vi "ClassPanel.vi"(8 "error in (no error)":errorcluster caption="entrée d'erreur (pas d'erreur)", 11 "TaikoLaser.lvclass":refnum<class "TaikoLaser.lvclass">) -> (0 "error out":errorcluster caption="sortie d'erreur", 3 "TaikoLaser.lvclass Out":refnum<class "TaikoLaser.lvclass">)   [LabVIEW 2019, in "TaikoLaser.lvclass"]
uses:
  TaikoLaser.lvclass
  <userlib>/TaikoLaser/PDLM_LaserMode.ctl
  C:/Programmes Labview/LabscanV1A/DevicesClass/BaseDevice/BaseDevice.lvclass
  <userlib>/TaikoLaser/PDLM_Tag.ctl
  <userlib>/TaikoLaser/PDLM_SystemStatus.ctl
  <userlib>/TaikoLaser/PDLM_TaggedValueList.ctl
  <userlib>/TaikoLaser/PDLM_TaggedValue.ctl
  TaikoLaser.lvclass/TaikoLaser.ctl
  BaseDevice/ClassQueueMess.ctl
  BaseDevice/BaseDevice.lvclass/BaseDevice.ctl
  <userlib>/TaikoLaser/PDLM_LaserLock.ctl
  BaseDevice/Accessor/GetBaseDataPath.vi
  BaseDevice/Accessor/GetClassEvent.vi
  <vilib>/Utility/error.llb/Error Cluster From Error Code.vi
  <vilib>/ErrorRing/Error Ring.xnode
panel:
  out "Error string":string
  out "ForceDis":bool caption="Force disconnect"
  out "Error":bool
  in  "UpdateCnter":u32
  out "JournalPath":path
  in  "Con/Disc.":bool
  out "InfoStr":string
  out "Shape String":string caption="Pulse Shape"
  out "Interlock":bool
  out "Temp":dbl caption="Temp (C)" min=0.1 step=0.1 format="%#.1f"
  out "updatedTag":T1[](array[typedef]) format="%x" items=["NONE"=0, "Locked"=16, "SoftLock"=17, "KeyLock"=18, "Class_IV_Lock"=20, "Interlock"=24, "LaserMode"=32, "LDH_PulsePowerTable"=33, "TriggerMode"=48, "TriggerLevelRaw"=64, "TriggerLevelRawLoLimit"=65, "TriggerLevelRawHiLimit"=66, "TriggerLevel"=72, "TriggerLevelLoLimit"=73, "TriggerLevelHiLimit"=74, "FastGate"=80, "FastGateImp"=96, "SlowGate"=112, "TargetTempRaw"=144, "TargetTempRawLoLimit"=145, "TargetTempRawHiLimit"=146, "CurrentTempRaw"=148, "CaseTempRaw"=149, "TargetTemp"=152, "TargetTempLoLimit"=153, "TargetTempHiLimit"=154, "CurrentTemp"=156, "CaseTemp"=157, "TempScale"=159, "Frequency"=168, "FrequencyLoLimit"=169, "FrequencyHiLimit"=170, "PulsePowerRaw"=176, "PulsePowerRawLoLimit"=177, "PulsePowerRawHiLimit"=178, "PulsePowerPermille"=180, "PulseShape"=181, "PulsePower"=184, "PulsePowerLoLimit"=185, "PulsePowerHiLimit"=186, "PulsePowerNanowatt"=188, "PulsePowerVoltage"=190, "PulseEnergy"=191, "CwPowerRaw"=192, "CwPowerRawLoLimit"=193, "CwPowerRawHiLimit"=194, "CwPowerPermille"=196, "CwPower"=200, "CwPowerLoLimit"=201, "CwPowerHiLimit"=202, "CwPowerMicroWatt"=204, "BurstLen"=208, "BurstPeriod"=224, "LDH_Fan"=240, "UI_Exclusive"=256]
  out "Act Power":dbl caption="Act. Power (mW)" min=0.1 step=0.1 format="%#.3f"
  in  "Update":bool
  in  "LaserMode":T2 caption="Laser Mode"
  in  "SoftLock":bool
  out "OnOffLock":bool
  out "KeyLock":bool
  in  "Power":dbl=0.1 caption="Output Power(%)" min=0.1 max=100.0 step=0.1 format="%#.1f"
  in  "MainProgQ":refnum<queue>
  in  "MainProgQEvent":refnum<user-event>
  in  "Acq":bool
  in  "Stop":bool
  in  "Frequ":dbl=50000.0 caption="Output Freq(kHz)" min=1.0 max=100000000.0 step=0.1 format="%#.1f"
  out "Init Program":bool
  # "Taiko Laser"
  # "this MUST labeled with class name"
  # "this MUST be present and labeled \"Stop\" and \"Acq\""
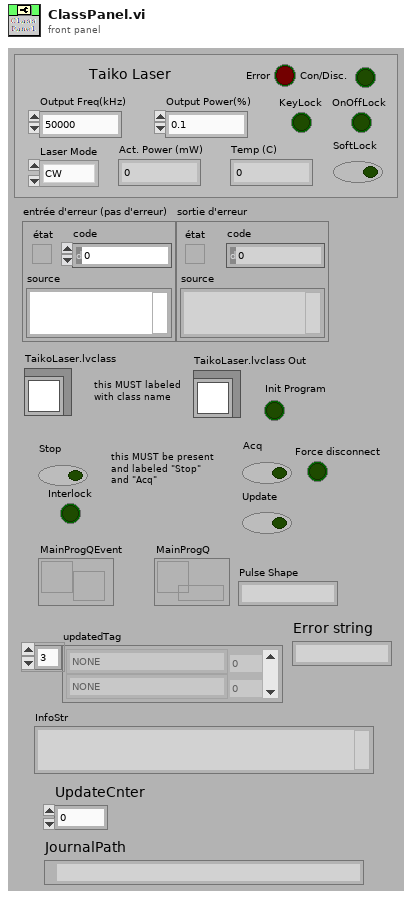
[diagram p1: front panel]
types:
  T1 = typedef "PDLM_Tag.ctl" = u32
  T2 = typedef "PDLM_LaserMode.ctl" = enum32{"CW", "PULSE", "BURST"}
  T3 = typedef "PDLM_SystemStatus.ctl" = u32
  T4 = typedef "PDLM_LaserLock.ctl" = enum32{"UNLOCKED", "LOCKED"}
  T5 = typedef "PDLM_TaggedValue.ctl" = cluster{"Tag":T1, "Value":u32}
  T6 = typedef "PDLM_TaggedValueList.ctl" = T5[]
  T7 = typedef "ClassQueueMess.ctl" = u16
  T8 = typedef "PDLM_LHInfo.ctl" = cluster{"LType":string, "Date":string, "LClass":string}
  T9 = typedef "PDLM_LHData.ctl" = cluster{"SerNo":u32, "Features":u32, "FreqMin":u32, "FreqMax":u32, "CwPowerMax":u32, "PulsePowerMax":u32, "WavelengthNominal":u16, "CaseTempMax":u16, "Protection":bool, "LHTypeCtrlVoltage":u16, "LHMaxVoltage":u16, "CurrentTEP12V":u16, "LaserType":T10, "LHVersion":T11, "CalWarrentHours":u16}
  T10 = typedef "PDLM_LHData_LaserType.ctl" = u16
  T11 = typedef "PDLM_LHVersion.ctl" = cluster{"Major":u16, "Minor":u16}
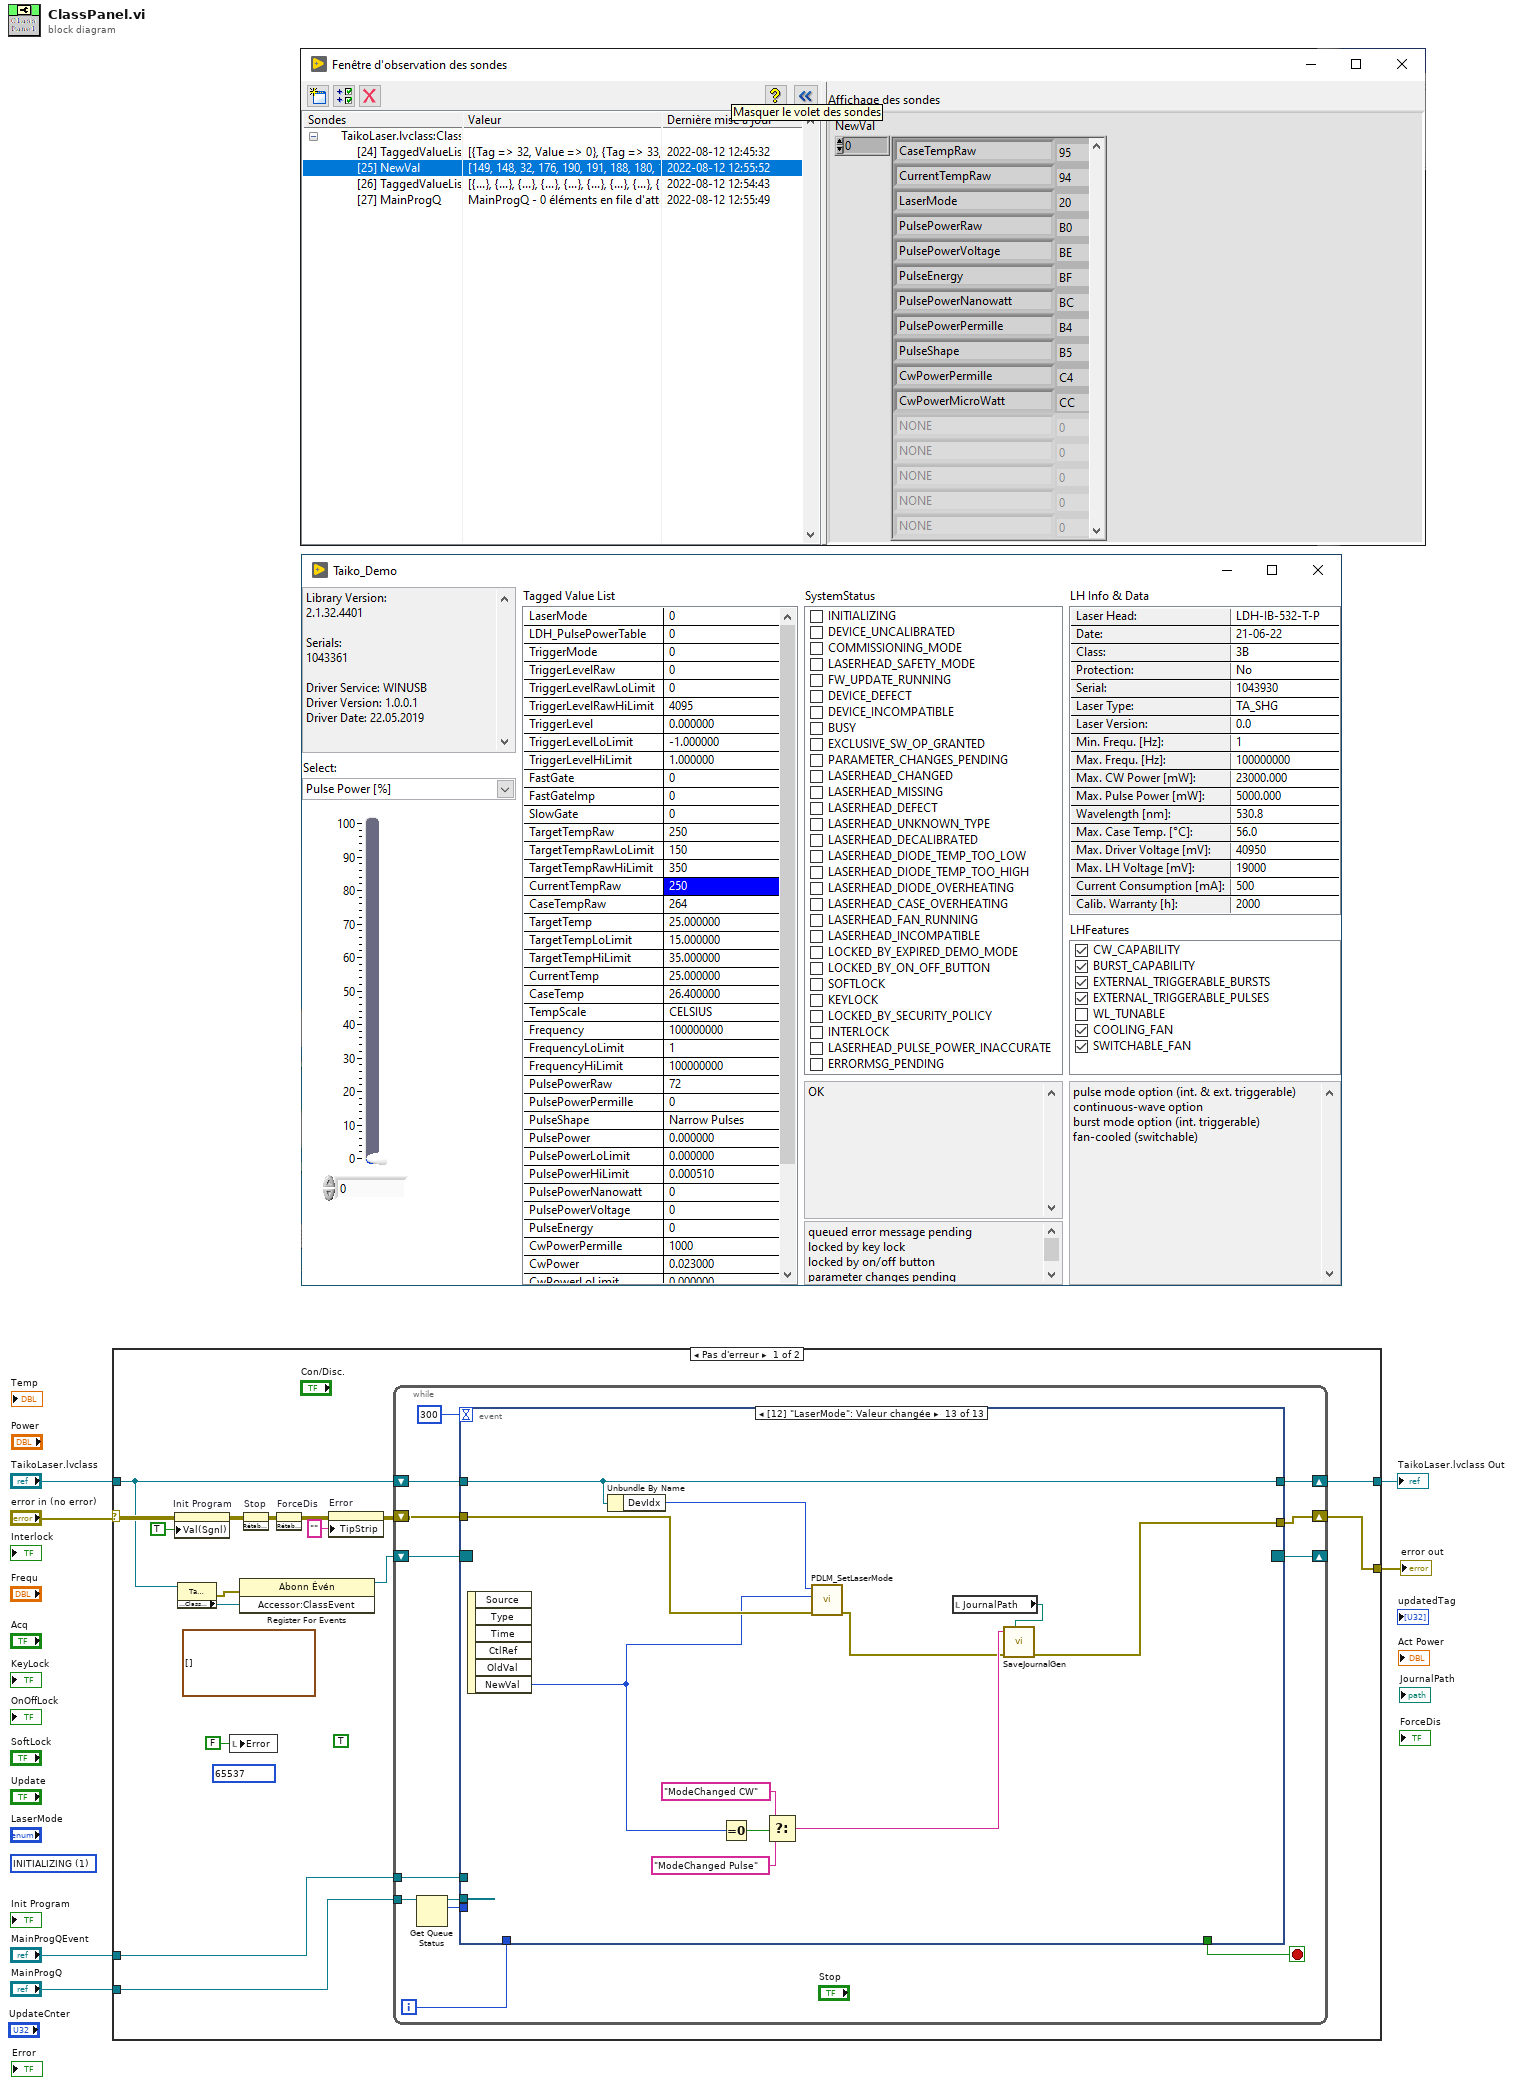
[diagram p0: block diagram]
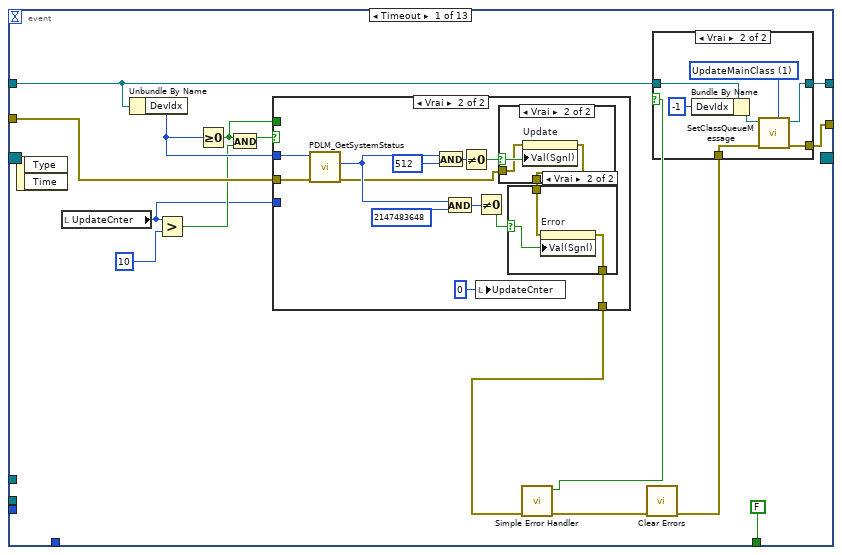
[diagram p2: hidden frame]
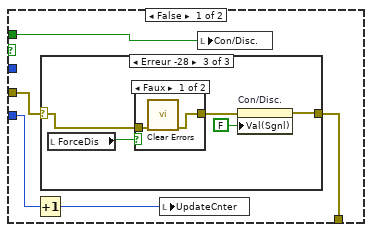
[diagram p4: hidden frame]
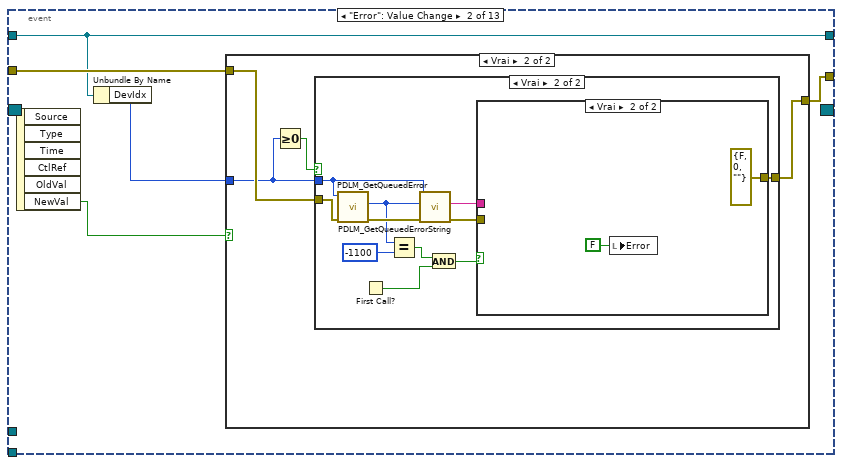
[diagram p10: hidden frame]
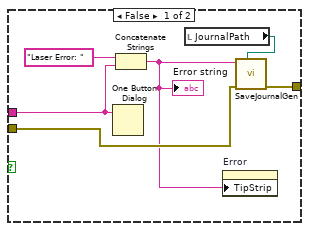
[diagram p13: hidden frame]
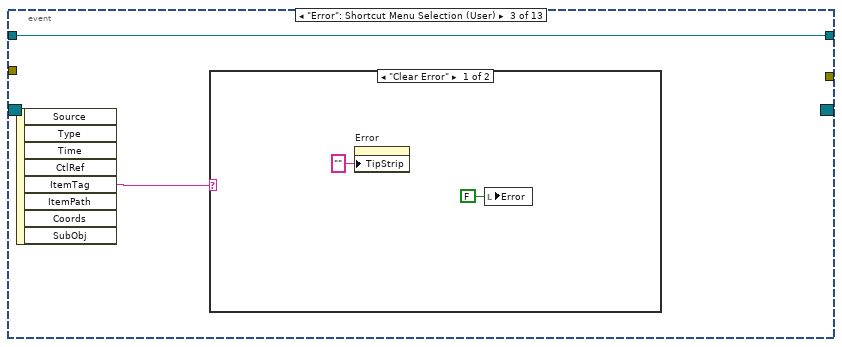
[diagram p14: hidden frame]
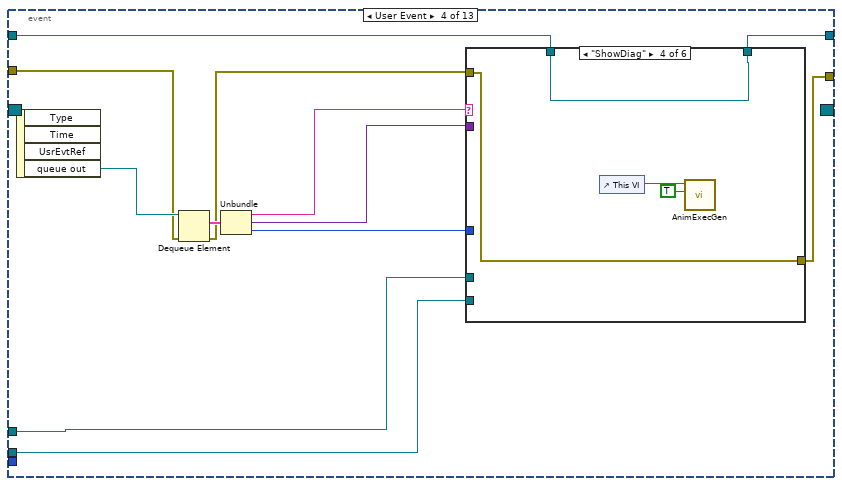
[diagram p16: hidden frame]
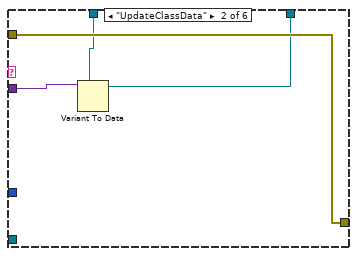
[diagram p18: hidden frame]
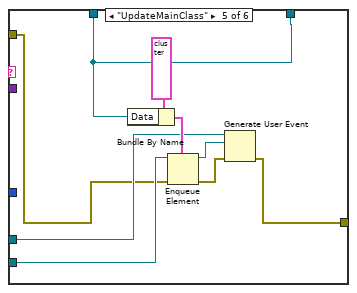
[diagram p20: hidden frame]
diagram:
  (unwired) T3 1 items=["INITIALIZING"=1, "DEVICE_UNCALIBRATED"=2, "COMMISSIONING_MODE"=4, "LASERHEAD_SAFETY_MODE"=8, "FW_UPDATE_RUNNING"=16, "DEVICE_DEFECT"=32, "DEVICE_INCOMPATIBLE"=64, "BUSY"=128, "EXCLUSIVE_SW_OP_GRANTED"=256, "PARAMETER_CHANGES_PENDING"=512, "LASERHEAD_CHANGED"=2048, "LASERHEAD_MISSING"=4096, "LASERHEAD_DEFECT"=8192, "LASERHEAD_UNKNOWN_TYPE"=16384, "LASERHEAD_DECALIBRATED"=32768, "LASERHEAD_DIODE_TEMP_TOO_LOW"=65536, "LASERHEAD_DIODE_TEMP_TOO_HIGH"=131072, "LASERHEAD_DIODE_OVERHEATING"=262144, "LASERHEAD_CASE_OVERHEATING"=524288, "LASERHEAD_FAN_RUNNING"=1048576, "LASERHEAD_INCOMPATIBLE"=2097152, "LOCKED_BY_EXPIRED_DEMO_MODE"=4194304, "LOCKED_BY_ON_OFF_BUTTON"=8388608, "SOFTLOCK"=16777216, "KEYLOCK"=33554432, "LOCKED_BY_SECURITY_POLICY"=67108864, "INTERLOCK"=134217728, "LASERHEAD_PULSE_POWER_INACCURATE"=268435456, "ERRORMSG_PENDING"=2147483648] ("SystemStatus")
  n1 = case shown="Pas d'erreur" "error in (no error)" {
    selector: "error in (no error)" -> [w11 w565]
    tunnel: [w22 w565] -> w5
    tunnel: "TaikoLaser.lvclass" -> [w16 w564]
    tunnel: [w20 w564] -> w3
    tunnel: "MainProgQEvent" -> [w14 _]
    tunnel: "MainProgQ" -> [w13 _]
    frame No Error {
      (unwired) TRUE ("ForceDis")
      (unwired) T1 65537 items=["NONE"=0, "Locked"=16, "SoftLock"=17, "KeyLock"=18, "Class_IV_Lock"=20, "Interlock"=24, "LaserMode"=32, "LDH_PulsePowerTable"=33, "TriggerMode"=48, "TriggerLevelRaw"=64, "TriggerLevelRawLoLimit"=65, "TriggerLevelRawHiLimit"=66, "TriggerLevel"=72, "TriggerLevelLoLimit"=73, "TriggerLevelHiLimit"=74, "FastGate"=80, "FastGateImp"=96, "SlowGate"=112, "TargetTempRaw"=144, "TargetTempRawLoLimit"=145, "TargetTempRawHiLimit"=146, "CurrentTempRaw"=148, "CaseTempRaw"=149, "TargetTemp"=152, "TargetTempLoLimit"=153, "TargetTempHiLimit"=154, "CurrentTemp"=156, "CaseTemp"=157, "TempScale"=159, "Frequency"=168, "FrequencyLoLimit"=169, "FrequencyHiLimit"=170, "PulsePowerRaw"=176, "PulsePowerRawLoLimit"=177, "PulsePowerRawHiLimit"=178, "PulsePowerPermille"=180, "PulseShape"=181, "PulsePower"=184, "PulsePowerLoLimit"=185, "PulsePowerHiLimit"=186, "PulsePowerNanowatt"=188, "PulsePowerVoltage"=190, "PulseEnergy"=191, "CwPowerRaw"=192, "CwPowerRawLoLimit"=193, "CwPowerRawHiLimit"=194, "CwPowerPermille"=196, "CwPower"=200, "CwPowerLoLimit"=201, "CwPowerHiLimit"=202, "CwPowerMicroWatt"=204, "BurstLen"=208, "BurstPeriod"=224, "LDH_Fan"=240, "UI_Exclusive"=256] ("Tag")
      (unwired) T6 [] ("TaggedValueList")
      n2 = property on="Init Program" class="Bool (strict)"(error in=w11, "Val(Sgnl)"=TRUE ("Valeur (Signalisation)")) -> (error out=w19:errorcluster)  [unwired: 1 in, 1 out]
      n3 = property class="TaikoLaser.lvclass"(reference=w16) -> (error out=w18:errorcluster, "Accessor:ClassEvent"=w17:refnum<user-event>)  [unwired: 1 in, 1 out]
      n4 = local write "Error"(FALSE ("Error")) -> ()
      n5 = register-events(error in=w18, w17) -> (reference out=w15:refnum<event-registration>)  [unwired: 1 in, 1 out]
      n6 = invoke on="Stop" class="Bool (strict)" method="RétablirValParDéfaut"(error in=w19) -> (error out=w10:errorcluster)  [unwired: 2 in, 2 out]
      n7 = invoke on="ForceDis" class="Bool (strict)" method="RétablirValParDéfaut"(error in=w10) -> (error out=w9:errorcluster)  [unwired: 2 in, 2 out]
      n8 = property on="Error" class="Bool (strict)"(error in=w9, "TipStrip"="" ("Info-bulle")) -> (error out=w8:errorcluster)  [unwired: 1 in, 1 out]
      n9 = while {
        shift-right: [w33] -> w22
        shift-left: w8 -> [w34]
        shift-right: [w32] -> w20
        shift-left: w16 -> [w26]
        shift-right: [w30] -> _
        shift-left: w15 -> [w31]
        tunnel: w14 -> [w29]
        tunnel: w13 -> [w28]
        i -> [w27]
        stop <- w25 stop-if-true
        n10 = Get Queue Status(queue=w28) -> (queue out=w24:refnum<queue>, # pending remove=w23:i32)  [unwired: 2 in, 6 out]
        n11 = event shown="[12] \"LaserMode\": Valeur changée" {
          selector: w31 -> [_ _ _ _ _ _ _ _ _ _ _ _ _]
          dyn-events: [_ _ _ _ _ _ _ _ _ _ _ _ _] -> w30
          timeout: 300 -> [_ _ _ _ _ _ _ _ _ _ _ _ _]
          tunnel: w34 -> [w48 w98 _ w131 w171 w208 w303 w317 w334 w354 w371 w415 w563]
          tunnel: [w42 w99 _ w135 w168 w213 w296 w313 w331 w345 w370 w409 w554] -> w33
          tunnel: w26 -> [w47 w97 w126 w141 w169 w211 w299 w316 w342 w357 w369 w412 w562]
          tunnel: [FALSE _ _ _ FALSE FALSE TRUE _ _ _ _ _ _] -> w25
          tunnel: [w45 w97 w126 w134 w167 w210 w299 w316 w342 w357 w368 w407 w562] -> w32
          tunnel: w29 -> [_ _ _ w133 _ _ _ _ _ _ _ _ _]
          tunnel: w24 -> [_ _ _ w132 _ _ _ _ _ _ _ _ _]
          tunnel: w27 -> [_ _ _ _ _ _ _ _ _ _ _ _ _]
          tunnel: w23 -> [_ _ _ _ _ _ _ _ _ _ _ _ _]
          event Timeout {
            n12 = event-data() -> ()  [unwired: 1 in, 2 out]
            n13 = local read "UpdateCnter"() -> (w38:u32)
            n14 = Unbundle By Name(w47) -> ("DevIdx"=w46:i32)
            n15 = Greater?(x=w38, y=u32 10) -> (0:w39:bool)
            n16 = Greater Or Equal To 0?(x=w46) -> (x >= 0?=w36:bool)
            n17 = And(x=w36, y=w39) -> (x .and. y?=w40:bool)
            n18 = case shown="Vrai" w40 {
              tunnel: w48 -> [w61 w87]
              tunnel: w46 -> [_ w86]
              tunnel: w38 -> [w64 _]
              tunnel: [w60 w75] -> w37
              tunnel: w36 -> [w62 _]
              frame False {
                n19 = Increment(x=w64) -> (x+1=w63:u32)
                n20 = case shown="Erreur -28" w61 {
                  selector: w61 -> [w65 w66 w70]
                  tunnel: [w65 w66 w68] -> w60
                  frame No Error {
                  }
                  frame Default {
                  }
                  frame Error {
                    n21 = local read "ForceDis"() -> (w71:bool)
                    n22 = case shown="Faux" w71 {
                      tunnel: w70 -> [w73 w74]
                      tunnel: [w72 w74] -> w69
                      frame False {
                        n23 = call <vilib>:"Clear Errors.vi"("error in (no error)"=w73) -> ("error out"=w72:errorcluster)  [unwired: 5 in, 1 out]
                      }
                      frame True {
                      }
                    }
                    n24 = property on="Con/Disc." class="Bool (strict)"(error in=w69, "Val(Sgnl)"=FALSE ("Valeur (Signalisation)")) -> (error out=w68:errorcluster)  [unwired: 1 in, 1 out]
                  }
                }
                n25 = local write "UpdateCnter"(w63) -> ()
                n26 = local write "Con/Disc."(w62) -> ()
              }
              frame True {
                n27 = call <userlib>:"PDLM_GetSystemStatus.vi"("error in (no error)"=w87, "USBIdx"=w86) -> ("error out"=w76:errorcluster, "state"=w82:u32)  [unwired: 7 in, 1 out]
                n28 = And(x=w82, y=u32 512) -> (x .and. y?=w81:u32)
                n29 = And(x=w82, y=u32 2147483648) -> (x .and. y?=w83:u32)
                n30 = Not Equal To 0?(x=w81) -> (x != 0?=w80:bool)
                n31 = Not Equal To 0?(x=w83) -> (x != 0?=w78:bool)
                n32 = local write "UpdateCnter"(u32 0 ("UpdateCnter")) -> ()
                n33 = case shown="Vrai" w80 {
                  selector: w80 -> [_ w95]
                  tunnel: [w92 w94] -> w77
                  tunnel: w76 -> [w92 w93]
                  frame False {
                  }
                  frame True {
                    n34 = property on="Update" class="Bool (strict)"(error in=w93, "Val(Sgnl)"=w95) -> (error out=w94:errorcluster)  [unwired: 1 in, 1 out]
                  }
                }
                n35 = case shown="Vrai" w78 {
                  selector: w78 -> [_ w91]
                  tunnel: w77 -> [w88 w90]
                  tunnel: [w88 w89] -> w75
                  frame False {
                  }
                  frame True {
                    n36 = property on="Error" class="Bool (strict)"(error in=w90, "Val(Sgnl)"=w91) -> (error out=w89:errorcluster)  [unwired: 1 in, 1 out]
                  }
                }
              }
            }
            n37 = call <vilib>:"Simple Error Handler.vi"("error in (no error)"=w37) -> ("error?"=w44:bool, "error out"=w49:errorcluster)  [unwired: 4 in, 3 out]
            n38 = call <vilib>:"Clear Errors.vi"("error in (no error)"=w49) -> ("error out"=w43:errorcluster)  [unwired: 5 in, 1 out]
            n39 = case shown="Vrai" w44 {
              tunnel: w47 -> [w52 w59]
              tunnel: [w52 w56] -> w45
              tunnel: w43 -> [w51 w54]
              tunnel: [w51 w53] -> w42
              frame False {
              }
              frame True {
                w55 = T7 1 items=["UpdateClassData", "UpdateMainClass", "UpdateDataBind"] ("Menu déroulant")
                n40 = Bundle By Name(cluster=w59, "DevIdx"=-1) -> (w57:refnum<class "TaikoLaser.lvclass">)
                n41 = call-dynamic "SetClassQueueMessage.vi"("ErrorIn(No Error)"=w54, "Menu déroulant"=w55, "DefaultDev.lvclass"=w57) -> ("sortie d'erreur"=w53:errorcluster, "DefaultDev.lvclass Out"=w56:refnum<class "TaikoLaser.lvclass">)  [unwired: 7 in]
              }
            }
          }
          event "Error": Value Change {
            n42 = event-data() -> ("NewVal"=w100:bool)  [unwired: 1 in, 5 out]
            n43 = Unbundle By Name(w97) -> ("DevIdx"=w96:i32)
            n44 = case shown="Vrai" w100 {
              tunnel: [w101 w104] -> w99
              tunnel: w98 -> [w101 w105]
              tunnel: w96 -> [_ w103]
              frame False {
              }
              frame True {
                n45 = Greater Or Equal To 0?(x=w103) -> (x >= 0?=w102:bool)
                n46 = case shown="Vrai" w102 {
                  tunnel: w103 -> [_ w116]
                  tunnel: w105 -> [w106 w115]
                  tunnel: [w106 w112] -> w104
                  frame False {
                  }
                  frame True {
                    n47 = call <userlib>:"PDLM_GetQueuedError.vi"("error in (no error)"=w115, "USBIdx"=w116) -> ("error out"=w117:errorcluster, "ErrCode"=w111:i32)  [unwired: 7 in, 1 out]
                    n48 = First Call?() -> (First Call?: T/F=w109:bool)
                    n49 = Equal?(x=w111, y=-1100) -> (x = y?=w108:bool)
                    n50 = call <userlib>:"PDLM_GetQueuedErrorString.vi"("error in (no error)"=w117, "ErrCode"=w111, "USBIdx"=w116) -> ("error out"=w113:errorcluster, "ErrText"=w114:string)  [unwired: 6 in, 1 out]
                    n51 = And(x=w108, y=w109) -> (x .and. y?=w107:bool)
                    n52 = case shown="Vrai" w107 {
                      tunnel: w114 -> [w122 _]
                      tunnel: w113 -> [w120 _]
                      tunnel: [w119 errorcluster {"status"=FALSE, "code"=0, "source"=""} ("error out")] -> w112
                      frame False {
                        n53 = One Button Dialog(message=w122) -> ()  [unwired: 1 in, 1 out]
                        n54 = Concatenate Strings("Laser Error: " ("chaîne"), w122) -> (w118:string)
                        "Error string" <- w118
                        n55 = local read "JournalPath"() -> (w123:path)
                        n56 = property on="Error" class="Bool (strict)"("TipStrip"=w118) -> ()  [unwired: 2 in, 2 out]
                        n57 = call <userlib>:"SaveJournalGen.vi"("CheminSauv"=w123, "error in"=w120, "Journal Text"=w118) -> ("error out"=w119:errorcluster)  [unwired: 7 in, 1 out]
                      }
                      frame True {
                        n58 = local write "Error"(FALSE ("Error")) -> ()
                      }
                    }
                  }
                }
              }
            }
          }
          event "Error": Shortcut Menu Selection (User) {
            n59 = event-data() -> ("ItemTag"=w127:string)  [unwired: 1 in, 7 out]
            n60 = case shown="\"Clear Error\"" w127 {
              frame "Clear Error" {
                n61 = property on="Error" class="Bool (strict)"("TipStrip"="" ("Info-bulle")) -> ()  [unwired: 2 in, 2 out]
                n62 = local write "Error"(FALSE ("Error")) -> ()
              }
              frame Default {
              }
            }
          }
          event User Event {
            n63 = event-data() -> ("queue out"=w139:refnum<queue>)  [unwired: 1 in, 3 out]
            n64 = Dequeue Element(queue=w139, error in (no error)=w131) -> (element=w140:cluster{"Message":string, "Data":variant, i32}, error out=w130:errorcluster)  [unwired: 1 in, 2 out]
            n65 = Unbundle(w140) -> ("Message"=w138:string, "Data"=w137:variant, w136:i32)
            n66 = case shown="\"ShowDiag\"" w138 {
              tunnel: w130 -> [w143 w147 w148 w152 w155 w165]
              tunnel: w137 -> [_ w146 _ _ _ _]
              tunnel: w141 -> [w142 w145 w149 w153 w158 w166]
              tunnel: [w142 w144 w149 w153 w158 w166] -> w134
              tunnel: [w143 w147 w148 w152 w154 w164] -> w135
              tunnel: w136 -> [_ _ _ _ _ _]
              tunnel: w133 -> [_ _ _ _ w157 _]
              tunnel: w132 -> [_ _ _ _ w156 _]
              frame Default {
              }
              frame "UpdateClassData" {
                n67 = Variant To Data(type=w145, Variant=w146) -> (data=w144:refnum<class "TaikoLaser.lvclass">)  [unwired: 1 in, 1 out]
              }
              frame "MeasDone" {
              }
              frame "ShowDiag" {
                n68 = control-ref of="This VI"() -> (w151:refnum<vi>)
                n69 = call <userlib>:"AnimExecGen.vi"("Animer l'exécution ?"=TRUE, "ViRef"=w151) -> ()  [unwired: 9 in, 1 out]
              }
              frame "UpdateMainClass" {
                n70 = Bundle By Name(cluster=cluster{"Message":string, "Data":variant, i32} {"Message"="", "Data"=variant, 0} ("élément"), "Data"=w158) -> (w159:cluster{"Message":string, "Data":variant, i32})
                n71 = Enqueue Element(queue=w156, element=w159, error in (no error)=w155) -> (queue out=w162:refnum<queue>, error out=w161:errorcluster)  [unwired: 1 in, 1 out]
                n72 = Generate User Event(user event=w157, event data cluster=w162, error in=w161) -> (error out=w154:errorcluster)  [unwired: 1 in, 1 out]
              }
              frame "ReInitDevice" {
                n73 = property on="Init Program" class="Bool (strict)"(error in=w165, "Val(Sgnl)"=TRUE ("Valeur (Signalisation)")) -> (error out=w164:errorcluster)  [unwired: 1 in, 1 out]
              }
            }
          }
          event "Con/Disc.": Value Change {
            n74 = event-data() -> ("NewVal"=w170:bool)  [unwired: 1 in]
            n75 = case shown="Faux" w170 {
              tunnel: w171 -> [w186 w204]
              tunnel: w169 -> [w182 w205]
              tunnel: [w178 w205] -> w167
              tunnel: [w177 w202] -> w168
              frame False {
                w180 = T7 1 items=["UpdateClassData", "UpdateMainClass", "UpdateDataBind"] ("Menu déroulant")
                n76 = Unbundle By Name(w182) -> ("DevIdx"=w185:i32)
                n77 = Greater Or Equal To 0?(x=w185) -> (x >= 0?=w184:bool)
                n78 = case shown="Faux" w184 {
                  tunnel: w186 -> [w191 w201]
                  tunnel: [w188 w200] -> w175
                  tunnel: w185 -> [_ w199]
                  tunnel: [w189 w198] -> w183
                  tunnel: w182 -> [w189 w198]
                  frame False {
                    n79 = local read "ForceDis"() -> (w187:bool)
                    n80 = case shown="Faux" w187 {
                      frame False {
                        n81 = property on="Init Program" class="Bool (strict)"("Val(Sgnl)"=TRUE ("Valeur (Signalisation)")) -> ()  [unwired: 2 in, 2 out]
                        n82 = local write "ForceDis"(TRUE ("ForceDis")) -> ()
                      }
                      frame True {
                      }
                    }
                    n83 = for {
                      N: 4 -> [_]
                      tunnel: w191 -> [w197]
                      tunnel: [w194] -> w188
                      tunnel: [w195] -> _
                      i -> [w196]
                      stop <- w194 continue-if-true
                      n84 = call <userlib>:"PDLM_CloseDevice.vi"("error in (no error)"=w197, "USBIdx"=w196) -> ("error out"=w194:errorcluster, "return type"=w195:i32)  [unwired: 8 in]
                    }
                  }
                  frame True {
                    n85 = call <userlib>:"PDLM_CloseDevice.vi"("error in (no error)"=w201, "USBIdx"=w199) -> ("error out"=w200:errorcluster)  [unwired: 8 in, 1 out]
                  }
                }
                n86 = Bundle By Name(cluster=w183, "DevIdx"=-1) -> (w179:refnum<class "TaikoLaser.lvclass">)
                n87 = local read "JournalPath"() -> (w176:path)
                n88 = call <userlib>:"SaveJournalGen.vi"("CheminSauv"=w176, "error in"=w175, "Journal Text"="TaikoSession Close") -> ("error out"=w174:errorcluster)  [unwired: 7 in, 1 out]
                n89 = call-dynamic "SetClassQueueMessage.vi"("ErrorIn(No Error)"=w174, "Menu déroulant"=w180, "DefaultDev.lvclass"=w179) -> ("sortie d'erreur"=w177:errorcluster, "DefaultDev.lvclass Out"=w178:refnum<class "TaikoLaser.lvclass">)  [unwired: 7 in]
              }
              frame True {
                n90 = property on="Init Program" class="Bool (strict)"(error in=w204, "Val(Sgnl)"=TRUE ("Valeur (Signalisation)")) -> (error out=w202:errorcluster)  [unwired: 1 in, 1 out]
              }
            }
          }
          event "Init Program": Value Change {
            n91 = event-data() -> ("NewVal"=w214:bool)  [unwired: 1 in]
            n92 = property class="TaikoLaser.lvclass"(reference=w211, error in=w208) -> (reference out=w209:refnum<class "TaikoLaser.lvclass">, error out=w207:errorcluster, "Accessor:BaseDataPath"=w206:path)
            n93 = case shown="Vrai" w214 {
              tunnel: w207 -> [w216 w232]
              tunnel: [w216 w248] -> w213
              tunnel: w209 -> [w215 w250]
              tunnel: [w215 w249] -> w210
              tunnel: w206 -> [_ w222]
              frame False {
              }
              frame True {
                w257 = T3 16777216 items=["INITIALIZING"=1, "DEVICE_UNCALIBRATED"=2, "COMMISSIONING_MODE"=4, "LASERHEAD_SAFETY_MODE"=8, "FW_UPDATE_RUNNING"=16, "DEVICE_DEFECT"=32, "DEVICE_INCOMPATIBLE"=64, "BUSY"=128, "EXCLUSIVE_SW_OP_GRANTED"=256, "PARAMETER_CHANGES_PENDING"=512, "LASERHEAD_CHANGED"=2048, "LASERHEAD_MISSING"=4096, "LASERHEAD_DEFECT"=8192, "LASERHEAD_UNKNOWN_TYPE"=16384, "LASERHEAD_DECALIBRATED"=32768, "LASERHEAD_DIODE_TEMP_TOO_LOW"=65536, "LASERHEAD_DIODE_TEMP_TOO_HIGH"=131072, "LASERHEAD_DIODE_OVERHEATING"=262144, "LASERHEAD_CASE_OVERHEATING"=524288, "LASERHEAD_FAN_RUNNING"=1048576, "LASERHEAD_INCOMPATIBLE"=2097152, "LOCKED_BY_EXPIRED_DEMO_MODE"=4194304, "LOCKED_BY_ON_OFF_BUTTON"=8388608, "SOFTLOCK"=16777216, "KEYLOCK"=33554432, "LOCKED_BY_SECURITY_POLICY"=67108864, "INTERLOCK"=134217728, "LASERHEAD_PULSE_POWER_INACCURATE"=268435456, "ERRORMSG_PENDING"=2147483648] ("SystemStatus")
                w264 = T3 33554432 items=["INITIALIZING"=1, "DEVICE_UNCALIBRATED"=2, "COMMISSIONING_MODE"=4, "LASERHEAD_SAFETY_MODE"=8, "FW_UPDATE_RUNNING"=16, "DEVICE_DEFECT"=32, "DEVICE_INCOMPATIBLE"=64, "BUSY"=128, "EXCLUSIVE_SW_OP_GRANTED"=256, "PARAMETER_CHANGES_PENDING"=512, "LASERHEAD_CHANGED"=2048, "LASERHEAD_MISSING"=4096, "LASERHEAD_DEFECT"=8192, "LASERHEAD_UNKNOWN_TYPE"=16384, "LASERHEAD_DECALIBRATED"=32768, "LASERHEAD_DIODE_TEMP_TOO_LOW"=65536, "LASERHEAD_DIODE_TEMP_TOO_HIGH"=131072, "LASERHEAD_DIODE_OVERHEATING"=262144, "LASERHEAD_CASE_OVERHEATING"=524288, "LASERHEAD_FAN_RUNNING"=1048576, "LASERHEAD_INCOMPATIBLE"=2097152, "LOCKED_BY_EXPIRED_DEMO_MODE"=4194304, "LOCKED_BY_ON_OFF_BUTTON"=8388608, "SOFTLOCK"=16777216, "KEYLOCK"=33554432, "LOCKED_BY_SECURITY_POLICY"=67108864, "INTERLOCK"=134217728, "LASERHEAD_PULSE_POWER_INACCURATE"=268435456, "ERRORMSG_PENDING"=2147483648] ("SystemStatus")
                w265 = T3 8388608 items=["INITIALIZING"=1, "DEVICE_UNCALIBRATED"=2, "COMMISSIONING_MODE"=4, "LASERHEAD_SAFETY_MODE"=8, "FW_UPDATE_RUNNING"=16, "DEVICE_DEFECT"=32, "DEVICE_INCOMPATIBLE"=64, "BUSY"=128, "EXCLUSIVE_SW_OP_GRANTED"=256, "PARAMETER_CHANGES_PENDING"=512, "LASERHEAD_CHANGED"=2048, "LASERHEAD_MISSING"=4096, "LASERHEAD_DEFECT"=8192, "LASERHEAD_UNKNOWN_TYPE"=16384, "LASERHEAD_DECALIBRATED"=32768, "LASERHEAD_DIODE_TEMP_TOO_LOW"=65536, "LASERHEAD_DIODE_TEMP_TOO_HIGH"=131072, "LASERHEAD_DIODE_OVERHEATING"=262144, "LASERHEAD_CASE_OVERHEATING"=524288, "LASERHEAD_FAN_RUNNING"=1048576, "LASERHEAD_INCOMPATIBLE"=2097152, "LOCKED_BY_EXPIRED_DEMO_MODE"=4194304, "LOCKED_BY_ON_OFF_BUTTON"=8388608, "SOFTLOCK"=16777216, "KEYLOCK"=33554432, "LOCKED_BY_SECURITY_POLICY"=67108864, "INTERLOCK"=134217728, "LASERHEAD_PULSE_POWER_INACCURATE"=268435456, "ERRORMSG_PENDING"=2147483648] ("SystemStatus")
                n94 = xnode "Menu déroulant d'erreurs"() -> ("sortie d'erreur"=w219:errorcluster)
                n95 = Not A Number/Path/Refnum?(number/path/refnum=w222) -> (NaN/Path/Refnum?=w225:bool)
                n96 = Empty String/Path?(string/path=w222) -> (empty?=w224:bool)
                n97 = call <userlib>:"PDLM_GetDLLPath.vi"("error in (no error)"=w232) -> ("error out"=w254:errorcluster)  [unwired: 8 in, 2 out]
                n98 = Or(x=w225, y=w224) -> (x .or. y?=w223:bool)
                n99 = for {
                  N: 8 -> [_]
                  tunnel: [w292] -> w251
                  tunnel: [w293] -> w218
                  tunnel: w254 -> [w294]
                  i -> [w292]
                  stop <- w293 continue-if-true
                  n100 = call <userlib>:"PDLM_OpenDevice.vi"("error in (no error)"=w294, "USBIdx"=w292) -> ("error out"=w293:errorcluster)  [unwired: 7 in, 2 out]
                }
                n101 = Select(t=path "c:/Data" ("cas vrai"), s=w223, f=w222) -> (s? t:f=w220:path)
                n102 = Build Path(base path=w220, name or relative path="TaikoLogs" ("nom ou chemin relatif")) -> (appended path=w229:path)
                n103 = File/Directory Info(path=w229) -> (error out=w230:errorcluster)  [unwired: 1 in, 6 out]
                n104 = Select(t=w219, s=w218, f=w218) -> (s? t:f=w217:errorcluster)
                n105 = case shown="Pas d'erreur" w230 {
                  selector: w230 -> [w273 _]
                  tunnel: w229 -> [w272 w276]
                  tunnel: [w273 w275] -> _
                  tunnel: [w272 w274] -> w228
                  frame No Error {
                  }
                  frame Error {
                    n106 = Create Folder(path (use dialog)=w276) -> (created path=w274:path, error out=w275:errorcluster)  [unwired: 2 in, 1 out]
                  }
                }
                n107 = Select(t=-1, s=w217, f=w251) -> (s? t:f=w245:i32)
                n108 = Build Path(base path=w228, name or relative path="TaikoLaserEvent.txt" ("nom ou chemin relatif")) -> (appended path=w226:path)
                n109 = local write "JournalPath"(w226) -> ()
                n110 = call <userlib>:"PDLM_GetSystemStatus.vi"("error in (no error)"=w217, "USBIdx"=w245) -> ("error out"=w259:errorcluster, "state"=w253:u32)  [unwired: 7 in, 1 out]
                n111 = And(x=w265, y=w253) -> (x .and. y?=w263:T3)
                n112 = And(x=w264, y=w253) -> (x .and. y?=w261:T3)
                n113 = call <userlib>:"PDLM_SetExclusiveUI.vi"("error in (no error)"=w259, "mode"=u32 0, "USBIdx"=w245) -> ("error out"=w244:errorcluster)  [unwired: 7 in, 1 out]
                n114 = call <userlib>:"PDLM_GetLHInfo.vi"("error in (no error)"=w244, "USBIdx"=w245) -> ("error out"=w246:errorcluster, "LHInfo"=w241:T8)  [unwired: 7 in, 1 out]
                n115 = call <userlib>:"PDLM_GetLHData.vi"("error in (no error)"=w246, "USBIdx"=w245) -> ("error out"=w243:errorcluster, "Data"=w242:T9)  [unwired: 7 in, 1 out]
                n116 = Unbundle By Name(w241) -> ("LType"=w240:string, "Date"=w239:string, "LClass"=w238:string)
                n117 = Not Equal To 0?(x=w263) -> (x != 0?=w262:bool)
                n118 = Not Equal To 0?(x=w261) -> (x != 0?=w260:bool)
                n119 = call <userlib>:"Taiko_LHDataToStrArray.vi"("LHData"=w242) -> ("StrArray"=w237:string[])  [unwired: 10 in]
                n120 = local write "OnOffLock"(w262) -> ()
                n121 = local write "KeyLock"(w260) -> ()
                n122 = Greater Or Equal To 0?(x=w245) -> (x >= 0?=w247:bool)
                n123 = Build Array (concatenate)(w240, w239, w238, w237) -> (w235:string[])
                n124 = case shown="Vrai" w247 {
                  selector: w247 -> [_ w287]
                  tunnel: [w283 w291] -> w248
                  tunnel: w243 -> [w283 w290]
                  tunnel: w226 -> [_ w288]
                  frame False {
                    n125 = local write "Init Program"(FALSE ("Init Program")) -> ()
                  }
                  frame True {
                    n126 = property on="Update" class="Bool (strict)"(error in=w290, "Val(Sgnl)"=w287) -> (error out=w291:errorcluster)  [unwired: 1 in, 1 out]
                    n127 = local write "Con/Disc."(TRUE ("Con/Disc.")) -> ()
                    n128 = local write "ForceDis"(FALSE ("ForceDis")) -> ()
                    n129 = call <userlib>:"SaveJournalGen.vi"("CheminSauv"=w288, "Journal Text"="LaserInit") -> ()  [unwired: 8 in, 2 out]
                  }
                }
                n130 = Bundle By Name(cluster=w250, "DevIdx"=w245) -> (w249:refnum<class "TaikoLaser.lvclass">)
                n131 = for {
                  tunnel: string[] ["Laser Head:", "Date:", "Class:", "Protection:", "Serial:", "Laser Type:", "Laser Version:", "Min. Frequ. [Hz]:", "Max. Frequ. [Hz]:", "Max. CW Power [mW]:", "Max. Pulse Power [mW]:", "Wavelength [nm]:", "Max. Case Temp. [°C]:", "Max. Driver Voltage [mV]:", "Max. LH Voltage [mV]:", "Current Consumption [mA]:", "Calib. Warranty [h]:"] ("Row Header Strings[]") -> [w282] mode=indexing
                  tunnel: w235 -> [w281] mode=indexing
                  shift-right: [w280] -> w233
                  shift-left: "" -> [w278]
                  n132 = call <vilib>:"Space Constant.vi"() -> ("String"=w277:string)
                  n133 = Concatenate Strings(w278, w282, w277, w281, "; " ("chaîne")) -> (w280:string)
                }
                "InfoStr" <- w233
                n134 = And(x=w257, y=w253) -> (x .and. y?=w258:T3)
                n135 = Not Equal To 0?(x=w258) -> (x != 0?=w256:bool)
                n136 = local write "SoftLock"(w256) -> ()
              }
            }
          }
          event "Stop": Value Change {
            n137 = event-data() -> ()  [unwired: 1 in, 5 out]
            n138 = Unbundle By Name(w299) -> ("DevIdx"=w300:i32)
            n139 = Greater Or Equal To 0?(x=w300) -> (x >= 0?=w301:bool)
            n140 = case shown="Vrai" w301 {
              tunnel: w300 -> [w304 w312]
              tunnel: w303 -> [w305 w311]
              tunnel: [w305 w310] -> w297
              frame False {
                # "try to close all idx"
                n141 = for {
                  N: 8 -> [_]
                  tunnel: w305 -> [w308]
                  tunnel: w304 -> [w307]
                  stop <- w309 continue-if-true
                  n142 = call <userlib>:"PDLM_CloseDevice.vi"("error in (no error)"=w308, "USBIdx"=w307) -> ("error out"=w309:errorcluster)  [unwired: 8 in, 1 out]
                }
              }
              frame True {
                n143 = call <userlib>:"PDLM_CloseDevice.vi"("error in (no error)"=w311, "USBIdx"=w312) -> ("error out"=w310:errorcluster)  [unwired: 8 in, 1 out]
              }
            }
            n144 = local read "JournalPath"() -> (w298:path)
            n145 = call <userlib>:"SaveJournalGen.vi"("CheminSauv"=w298, "error in"=w297, "Journal Text"="TaikoPanel Closed") -> ("error out"=w296:errorcluster)  [unwired: 7 in, 1 out]
          }
          event "SoftLock": Value Change {
            n146 = event-data() -> ("NewVal"=w320:bool)  [unwired: 1 in]
            n147 = Select(t=PDLM_LaserLock."LOCKED" ("SoftLocked"), s=w320, f=PDLM_LaserLock."UNLOCKED" ("SoftLocked")) -> (s? t:f=w318:T4)
            n148 = Unbundle By Name(w316) -> ("DevIdx"=w314:i32)
            n149 = Greater Or Equal To 0?(x=w314) -> (x >= 0?=w315:bool)
            n150 = case shown="Vrai" w315 {
              tunnel: w318 -> [_ w327]
              tunnel: w317 -> [w322 w330]
              tunnel: w314 -> [_ w329]
              tunnel: [w322 w324] -> w313
              frame False {
              }
              frame True {
                n151 = call <userlib>:"PDLM_SetSoftLock.vi"("error in (no error)"=w330, "SoftLocked"=w327, "USBIdx"=w329) -> ("error out"=w326:errorcluster)  [unwired: 7 in, 1 out]
                n152 = local read "JournalPath"() -> (w323:path)
                n153 = Format Into String(format string="SetSoftLock %d" ("chaîne de format"), w327) -> (resulting string=w325:string)  [unwired: 2 in, 1 out]
                n154 = call <userlib>:"SaveJournalGen.vi"("CheminSauv"=w323, "error in"=w326, "Journal Text"=w325) -> ("error out"=w324:errorcluster)  [unwired: 7 in, 1 out]
              }
            }
          }
          event "Frequ": Value Change {
            n155 = event-data() -> ("NewVal"=w341:dbl)  [unwired: 1 in]
            n156 = Multiply(x=1000.0, y=w341) -> (x*y=w340:dbl)
            n157 = Unbundle By Name(w342) -> ("DevIdx"=w343:i32)
            n158 = To Unsigned Long Integer(number=w340) -> (unsigned 32bit integer=w338:u32)
            n159 = call <userlib>:"PDLM_SetFrequency.vi"("error in (no error)"=w334, "freq"=w338, "USBIdx"=w343) -> ("error out"=w333:errorcluster)  [unwired: 7 in, 1 out]
            n160 = Format Into String(format string="SetFrequency %d Hz" ("chaîne de format"), error in=w333, w338) -> (resulting string=w336:string, error out=w332:errorcluster)  [unwired: 1 in]
            n161 = local read "JournalPath"() -> (w335:path)
            n162 = call <userlib>:"SaveJournalGen.vi"("CheminSauv"=w335, "error in"=w332, "Journal Text"=w336) -> ("error out"=w331:errorcluster)  [unwired: 7 in, 1 out]
          }
          event "Power": Value Change {
            n163 = event-data() -> ("NewVal"=w352:dbl)  [unwired: 1 in]
            n164 = Unbundle By Name(w357) -> ("DevIdx"=w356:i32)
            n165 = local read "LaserMode"() -> (w355:T2)
            n166 = Multiply(x=10.0, y=w352) -> (x*y=w353:dbl)
            n167 = To Unsigned Long Integer(number=w353) -> (unsigned 32bit integer=w350:u32)
            n168 = case shown="\"CW\", Par défaut" w355 {
              tunnel: w356 -> [w360 w367]
              tunnel: w354 -> [w362 w366]
              tunnel: w350 -> [w361 w365]
              tunnel: ["SetCWPower %d %" ("chaîne de format") "SetPulsePower %d %" ("chaîne de format")] -> w347
              tunnel: [w359 w363] -> w346
              frame "CW", Default {
                n169 = call <userlib>:"PDLM_SetCwPowerPermille.vi"("error in (no error)"=w362, "permille"=w361, "USBIdx"=w360) -> ("error out"=w359:errorcluster)  [unwired: 7 in, 1 out]
              }
              frame "PULSE" {
                n170 = call <userlib>:"PDLM_SetPulsePowerPermille.vi"("error in (no error)"=w366, "permille"=w365, "USBIdx"=w367) -> ("error out"=w363:errorcluster)  [unwired: 7 in, 1 out]
              }
            }
            n171 = Format Into String(format string=w347, error in=w346, w350) -> (resulting string=w348:string, error out=w349:errorcluster)  [unwired: 1 in]
            n172 = local read "JournalPath"() -> (w344:path)
            n173 = call <userlib>:"SaveJournalGen.vi"("CheminSauv"=w344, "error in"=w349, "Journal Text"=w348) -> ("error out"=w345:errorcluster)  [unwired: 7 in, 1 out]
          }
          event "Update": Value Change {
            n174 = event-data() -> ()  [unwired: 1 in, 5 out]
            n175 = local read "Init Program"() -> (w372:bool)
            n176 = Unbundle By Name(w369) -> ("DevIdx"=w373:i32)
            n177 = case shown="Faux" w372 {
              tunnel: w373 -> [w380 w401]
              tunnel: w371 -> [w379 w399]
              tunnel: [w381 w396] -> w370
              tunnel: w369 -> [w375 w394]
              tunnel: [w374 w393] -> w368
              frame False {
                n178 = call <userlib>:"GetEmptyTagValueList.vi"("error in (no error)"=w379) -> ("error out"=w383:errorcluster, "Array"=w382:T5[])  [unwired: 9 in]
                n179 = call <userlib>:"PDLM_GetQueuedChanges.vi"("error in (no error)"=w383, "TaggedValueList"=w382, "USBIdx"=w380) -> ("error out"=w381:errorcluster, "ListLen out"=w377:u32, "TaggedValueList out"=w378:T6)  [unwired: 5 in, 1 out]
                n180 = Greater Than 0?(x=w377) -> (x > 0?=w376:bool)
                n181 = case shown="Vrai" w376 {
                  tunnel: w378 -> [_ w386]
                  tunnel: w377 -> [_ w388]
                  tunnel: w375 -> [w384 w387]
                  tunnel: [w384 w385] -> w374
                  frame False {
                  }
                  frame True {
                    n182 = for {
                      N: w388 -> [_]
                      tunnel: w386 -> [w391] mode=indexing
                      tunnel: [w390] -> w389 mode=indexing
                      n183 = Unbundle By Name(w391) -> ("Tag"=w390:T1)
                    }
                    n184 = Bundle By Name(cluster=w387, "TaggedValueList"=w386) -> (w385:refnum<class "TaikoLaser.lvclass">)
                    n185 = property on="updatedTag" class="Tabl (strict)"("Val(Sgnl)"=w389) -> ()  [unwired: 2 in, 2 out]
                  }
                }
              }
              frame True {
                (unwired) TRUE
                n186 = local write "Init Program"(FALSE ("Init Program")) -> ()
                n187 = local write "Con/Disc."(TRUE ("Init Program")) -> ()
                n188 = call <userlib>:"PDLM_GetTagValueList.vi"("error in (no error)"=w399, "TaggedValueList"=T5[] [{"Tag"=32, "Value"=0}, {"Tag"=33, "Value"=0}, {"Tag"=48, "Value"=0}, {"Tag"=64, "Value"=0}, {"Tag"=65, "Value"=0}, {"Tag"=66, "Value"=0}, {"Tag"=72, "Value"=0}, {"Tag"=73, "Value"=0}, {"Tag"=74, "Value"=0}, {"Tag"=80, "Value"=0}, {"Tag"=96, "Value"=0}, {"Tag"=112, "Value"=0}, {"Tag"=144, "Value"=0}, {"Tag"=145, "Value"=0}, {"Tag"=146, "Value"=0}, {"Tag"=148, "Value"=0}, {"Tag"=149, "Value"=0}, {"Tag"=152, "Value"=0}, {"Tag"=153, "Value"=0}, {"Tag"=154, "Value"=0}, {"Tag"=156, "Value"=0}, {"Tag"=157, "Value"=0}, {"Tag"=159, "Value"=0}, {"Tag"=168, "Value"=0}, {"Tag"=169, "Value"=0}, {"Tag"=170, "Value"=0}, {"Tag"=176, "Value"=0}, {"Tag"=180, "Value"=0}, {"Tag"=181, "Value"=0}, {"Tag"=184, "Value"=0}, {"Tag"=185, "Value"=0}, {"Tag"=186, "Value"=0}, {"Tag"=188, "Value"=0}, {"Tag"=190, "Value"=0}, {"Tag"=191, "Value"=0}, {"Tag"=196, "Value"=0}, {"Tag"=200, "Value"=0}, {"Tag"=201, "Value"=0}, {"Tag"=202, "Value"=0}, {"Tag"=204, "Value"=0}, {"Tag"=208, "Value"=0}, {"Tag"=224, "Value"=0}, {"Tag"=240, "Value"=0}, {"Tag"=256, "Value"=0}] ("Tableau"), "USBIdx"=w401) -> ("error out"=w397:errorcluster, "TaggedValueList out"=w395:T6)  [unwired: 6 in, 1 out]
                n189 = for {
                  tunnel: w395 -> [w404] mode=indexing
                  tunnel: [w403] -> w398 mode=indexing
                  n190 = Unbundle By Name(w404) -> ("Tag"=w403:T1)
                }
                n191 = Bundle By Name(cluster=w394, "TaggedValueList"=w395) -> (w393:refnum<class "TaikoLaser.lvclass">)
                n192 = property on="updatedTag" class="Tabl (strict)"(error in=w397, "Val(Sgnl)"=w398) -> (error out=w396:errorcluster)  [unwired: 1 in, 1 out]
              }
            }
          }
          event "updatedTag": Value Change {
            w411 = T7 1 items=["UpdateClassData", "UpdateMainClass", "UpdateDataBind"] ("Menu déroulant")
            n193 = event-data() -> ("NewVal"=w413:T1[])  [unwired: 1 in, 5 out]
            n194 = Unbundle By Name(w412) -> ("TaggedValueList"=w414:T6)
            n195 = local read "Init Program"() -> (w406:bool)
            n196 = for {
              shift-right: [w419] -> w410
              shift-left: w415 -> [w426]
              tunnel: w414 -> [w425] mode=indexing
              tunnel: w413 -> [_] mode=indexing
              shift-right: [w421] -> w408
              shift-left: w412 -> [w422]
              tunnel: w406 -> [w417]
              tunnel: [w416] -> w405
              (unwired) T1 191 items=["NONE"=0, "Locked"=16, "SoftLock"=17, "KeyLock"=18, "Class_IV_Lock"=20, "Interlock"=24, "LaserMode"=32, "LDH_PulsePowerTable"=33, "TriggerMode"=48, "TriggerLevelRaw"=64, "TriggerLevelRawLoLimit"=65, "TriggerLevelRawHiLimit"=66, "TriggerLevel"=72, "TriggerLevelLoLimit"=73, "TriggerLevelHiLimit"=74, "FastGate"=80, "FastGateImp"=96, "SlowGate"=112, "TargetTempRaw"=144, "TargetTempRawLoLimit"=145, "TargetTempRawHiLimit"=146, "CurrentTempRaw"=148, "CaseTempRaw"=149, "TargetTemp"=152, "TargetTempLoLimit"=153, "TargetTempHiLimit"=154, "CurrentTemp"=156, "CaseTemp"=157, "TempScale"=159, "Frequency"=168, "FrequencyLoLimit"=169, "FrequencyHiLimit"=170, "PulsePowerRaw"=176, "PulsePowerRawLoLimit"=177, "PulsePowerRawHiLimit"=178, "PulsePowerPermille"=180, "PulseShape"=181, "PulsePower"=184, "PulsePowerLoLimit"=185, "PulsePowerHiLimit"=186, "PulsePowerNanowatt"=188, "PulsePowerVoltage"=190, "PulseEnergy"=191, "CwPowerRaw"=192, "CwPowerRawLoLimit"=193, "CwPowerRawHiLimit"=194, "CwPowerPermille"=196, "CwPower"=200, "CwPowerLoLimit"=201, "CwPowerHiLimit"=202, "CwPowerMicroWatt"=204, "BurstLen"=208, "BurstPeriod"=224, "LDH_Fan"=240, "UI_Exclusive"=256] ("Tag")
              # "cwpowerPermille"
              n197 = Unbundle By Name(w425) -> ("Tag"=w424:T1, "Value"=w423:u32)
              n198 = case shown="196" w424 {
                selector: w424 -> [w436 _ _ _ _ _ _ _ _ _ _ _ _ _ _]
                tunnel: [w439 w444 w450 w456 w462 w478 w486 w491 w500 w505 w514 w521 w526 w535 w545] -> w420
                tunnel: w426 -> [w439 w444 w450 w456 w463 w478 w486 w491 w500 w505 w514 w521 w526 w535 w545]
                tunnel: w423 -> [w435 w442 w447 w453 w469 w477 w481 w488 w493 w504 w508 w518 w524 w528 w539]
                tunnel: [_ _ _ _ _ _ _ w488 _ _ _ _ w524 _ _] -> _
                tunnel: w422 -> [w438 w443 w449 w455 w470 w474 w482 w490 w495 w503 w509 w520 w525 w530 w540]
                tunnel: [w438 w443 w449 w455 w461 w474 w482 w490 w495 w503 w509 w520 w525 w530 w540] -> w421
                tunnel: [w434 w440 w446 w452 w458 w471 w479 w487 w492 w502 w506 w517 w522 w527 w538] -> w418
                frame 0, Default {
                  n199 = Format Into String(format string="Unknown tag# %d; Val: %d", w436, w435) -> (resulting string=w434:string)  [unwired: 2 in, 1 out]
                }
                frame 17 {
                  n200 = Not Equal To 0?(x=w442) -> (x != 0?=w445:bool)
                  n201 = local write "SoftLock"(w445) -> ()
                  n202 = Format Into String(format string="SoftLock %d" ("chaîne de format"), w442) -> (resulting string=w440:string)  [unwired: 2 in, 1 out]
                }
                frame 18 {
                  n203 = Not Equal To 0?(x=w447) -> (x != 0?=w451:bool)
                  n204 = local write "KeyLock"(w451) -> ()
                  n205 = Format Into String(format string="KeyLock %d" ("chaîne de format"), w447) -> (resulting string=w446:string)  [unwired: 2 in, 1 out]
                }
                frame 24 {
                  n206 = Not Equal To 0?(x=w453) -> (x != 0?=w457:bool)
                  n207 = local write "Interlock"(w457) -> ()
                  n208 = Format Into String(format string="InterLock %d" ("chaîne de format"), w453) -> (resulting string=w452:string)  [unwired: 2 in, 1 out]
                }
                frame 32 {
                  n209 = Equal To 0?(x=w469) -> (x = 0?=w468:bool)
                  n210 = Select(t="CW Power(W)", s=w468, f="Pulse Power(W)") -> (s? t:f=w460:string)
                  n211 = Build Array("OutputPower(%)", w460) -> (w464:string[])
                  n212 = property class="TaikoLaser.lvclass"(reference=w470, error in=w463, "Accessor:DataNames"=w464) -> (reference out=w461:refnum<class "TaikoLaser.lvclass">, error out=w462:errorcluster)
                  n213 = Concatenate Strings("Mode Changed :" ("chaîne"), w460) -> (w458:string)
                  n214 = local write "LaserMode"(w469) -> ()
                }
                frame 148 {
                  # "CurrentTempRaw"
                  n215 = To Double Precision Float(number=w477) -> (double precision float=w476:dbl)
                  n216 = Divide(x=w476, y=10.0) -> (x/y=w473:dbl)
                  n217 = local write "Temp"(w473) -> ()
                  n218 = Format Into String(format string="Temp %.2f C" ("chaîne de format"), w473) -> (resulting string=w471:string)  [unwired: 2 in, 1 out]
                }
                frame 168 {
                  n219 = To Double Precision Float(number=w481) -> (double precision float=w484:dbl)
                  n220 = Divide(x=w484, y=1000.0) -> (x/y=w485:dbl)
                  n221 = local write "Frequ"(w485) -> ()
                  n222 = Format Into String(format string="Freq Changed %d Hz" ("chaîne de format"), w481) -> (resulting string=w479:string)  [unwired: 2 in, 1 out]
                }
                frame 176 {
                  # "pulsepowerraw"
                  n223 = Format Into String(format string="pulsepowerraw %d" ("Buffer"), w488) -> (resulting string=w487:string)  [unwired: 2 in, 1 out]
                }
                frame 180 {
                  # "PulsepowerPermille"
                  n224 = local read "LaserMode"() -> (w496:T2)
                  n225 = To Double Precision Float(number=w493) -> (double precision float=w499:dbl)
                  n226 = Divide(x=w499, y=10.0) -> (x/y=w497:dbl)
                  n227 = Format Into String(format string="PulsepowerPermille %d" ("Buffer"), w493) -> (resulting string=w492:string)  [unwired: 2 in, 1 out]
                  n228 = case shown="\"PULSE\"" w496 {
                    tunnel: w497 -> [_ w501]
                    frame "CW", Default {
                    }
                    frame "PULSE" {
                      n229 = local write "Power"(w501) -> ()
                    }
                  }
                }
                frame 181 {
                  # "PulseShape"
                  n230 = call <userlib>:"PDLM_DecodePulseShape.vi"("shape"=w504) -> ("Buffer"=w502:string)  [unwired: 8 in, 2 out]
                  "Shape String" <- w502
                }
                frame 188 {
                  # "PulsePowerNanowatt"
                  n231 = local read "LaserMode"() -> (w510:T2)
                  n232 = To Double Precision Float(number=w508) -> (double precision float=w513:dbl)
                  n233 = Divide(x=w513, y=1000.0) -> (x/y=w511:dbl)
                  n234 = case shown="\"PULSE\"" w510 {
                    tunnel: w511 -> [_ w516]
                    frame "CW", Default {
                    }
                    frame "PULSE" {
                      n235 = local write "Act Power"(w516) -> ()
                      n236 = property on="Act Power" class="NumNb (strict)"("Caption.Text"="Pulse Power (uW)" ("Sous-titre.Texte")) -> ()  [unwired: 2 in, 2 out]
                    }
                  }
                  n237 = Format Into String(initial string="PulsePowerNanowatt %d" ("Buffer"), w508) -> (resulting string=w506:string)  [unwired: 2 in, 1 out]
                }
                frame 191 {
                  # "PulseEnergy"
                  n238 = Format Into String(format string="PulseEnergy %d" ("Buffer"), w518) -> (resulting string=w517:string)  [unwired: 2 in, 1 out]
                }
                frame 192 {
                  # "cwpowerraw"
                  n239 = Format Into String(format string="cwpowerraw %d" ("Buffer"), w524) -> (resulting string=w522:string)  [unwired: 2 in, 1 out]
                }
                frame 204 {
                  # "cwpowermicrowatt"
                  n240 = To Double Precision Float(number=w528) -> (double precision float=w534:dbl)
                  n241 = local read "LaserMode"() -> (w531:T2)
                  n242 = Divide(x=w534, y=1000.0) -> (x/y=w532:dbl)
                  n243 = case shown="\"CW\"" w531 {
                    tunnel: w532 -> [w537 _]
                    frame "CW" {
                      n244 = local write "Act Power"(w537) -> ()
                      n245 = property on="Act Power" class="NumNb (strict)"("Caption.Text"="CW Power (mW)" ("Sous-titre.Texte")) -> ()  [unwired: 2 in, 2 out]
                    }
                    frame "PULSE", Default {
                    }
                  }
                  n246 = Format Into String(format string="cwpowermicrowatt %d" ("Buffer"), w528) -> (resulting string=w527:string)  [unwired: 2 in, 1 out]
                }
                frame 196 {
                  # "cwpowerPermille"
                  n247 = To Double Precision Float(number=w539) -> (double precision float=w544:dbl)
                  n248 = local read "LaserMode"() -> (w541:T2)
                  n249 = Divide(x=w544, y=10.0) -> (x/y=w542:dbl)
                  n250 = case shown="\"PULSE\", Par défaut" w541 {
                    tunnel: w542 -> [w549 _]
                    tunnel: w539 -> [w548 w552]
                    tunnel: [w546 w550] -> w538
                    frame "CW" {
                      n251 = local write "Power"(w549) -> ()
                      n252 = Format Into String(format string="CWPowerChanged %d %" ("chaîne de format"), w548) -> (resulting string=w546:string)  [unwired: 2 in, 1 out]
                    }
                    frame "PULSE", Default {
                      n253 = Format Into String(initial string="PulsePowerChanged %d %" ("chaîne de format"), w552) -> (resulting string=w550:string)  [unwired: 2 in, 1 out]
                    }
                  }
                }
              }
              n254 = case shown="Vrai" w417 {
                tunnel: w420 -> [w428 w432]
                tunnel: [w428 w431] -> w419
                tunnel: w418 -> [_ w430]
                tunnel: [FALSE FALSE] -> w416
                frame False {
                }
                frame True {
                  n255 = local read "JournalPath"() -> (w433:path)
                  n256 = call <userlib>:"SaveJournalGen.vi"("CheminSauv"=w433, "error in"=w432, "Journal Text"=w430) -> ("error out"=w431:errorcluster)  [unwired: 7 in, 1 out]
                }
              }
            }
            n257 = local write "Init Program"(w405) -> ()
            n258 = call-dynamic "SetClassQueueMessage.vi"("ErrorIn(No Error)"=w410, "Menu déroulant"=w411, "DefaultDev.lvclass"=w408) -> ("sortie d'erreur"=w409:errorcluster, "DefaultDev.lvclass Out"=w407:refnum<class "TaikoLaser.lvclass">)  [unwired: 7 in]
          }
          event Value Change {
            n259 = event-data() -> ("NewVal"=w553:T2)  [unwired: 1 in, 5 out]
            n260 = Unbundle By Name(w562) -> ("DevIdx"=w561:i32)
            n261 = Equal To 0?(x=w553) -> (x = 0?=w559:bool)
            n262 = Select(t="ModeChanged CW" ("chaîne de format"), s=w559, f="ModeChanged Pulse" ("chaîne de format")) -> (s? t:f=w556:string)
            n263 = call <userlib>:"PDLM_SetLaserMode.vi"("error in (no error)"=w563, "mode"=w553, "USBIdx"=w561) -> ("error out"=w555:errorcluster)  [unwired: 7 in, 1 out]
            n264 = local read "JournalPath"() -> (w560:path)
            n265 = call <userlib>:"SaveJournalGen.vi"("CheminSauv"=w560, "error in"=w555, "Journal Text"=w556) -> ("error out"=w554:errorcluster)  [unwired: 7 in, 1 out]
          }
        }
      }
    }
    frame Error {
    }
  }
  "error out" <- w5
  "TaikoLaser.lvclass Out" <- w3
